vi "tankdrive.vi"(9 "Right Value":dbl, 10 "Left Value":dbl) -> ()   [LabVIEW 2013]
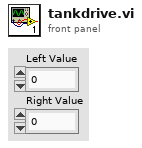
[diagram p1: front panel]
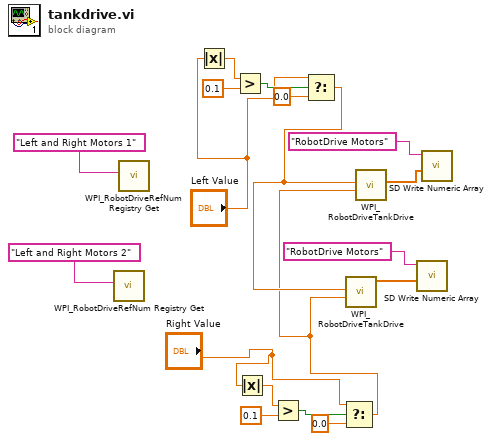
[diagram p0: block diagram]
diagram:
  n1 = call <vilib>:"WPI_RobotDriveRefNum Registry Get.vi"("refnum name"="Left and Right Motors 2") -> ()  [unwired: 1 in, 10 out]
  n2 = call <vilib>:"WPI_RobotDriveRefNum Registry Get.vi"("refnum name"="Left and Right Motors 1") -> ()  [unwired: 1 in, 10 out]
  n3 = Absolute Value(x="Left Value") -> (abs(x)=w4:dbl)
  n4 = Greater?(x=w4, y=0.1) -> (0:w6:bool)
  n5 = Absolute Value(x="Right Value") -> (abs(x)=w10:dbl)
  n6 = Greater?(x=w10, y=0.1) -> (0:w13:bool)
  n7 = Select(t="Left Value", s=w6, f=0.0) -> (s? t:f=w2:dbl)
  n8 = Select(t="Right Value", s=w13, f=0.0) -> (s? t:f=w1:dbl)
  n9 = call <vilib>:"WPI_RobotDriveTankDrive.vi"("Right axis value"=w1, "Left axis value"=w2) -> ("Motor Values"=w9:dbl[])  [unwired: 7 in, 2 out]
  n10 = call <vilib>:"WPI_RobotDriveTankDrive.vi"("Right axis value"=w1, "Left axis value"=w2) -> ("Motor Values"=w8:dbl[])  [unwired: 7 in, 2 out]
  n11 = call <vilib>:"SD Write Numeric Array.vi"("Numeric Array"=w9, "Name"="RobotDrive Motors") -> ()  [unwired: 8 in, 2 out]
  n12 = call <vilib>:"SD Write Numeric Array.vi"("Numeric Array"=w8, "Name"="RobotDrive Motors") -> ()  [unwired: 8 in, 2 out]
